vi "ELVIS III v1.0 AI Continuous Read.vi"(5 "Timeout":i32=-1 min=-1, 7 "Number of Samples":u32, 8 "error in (no error)":errorcluster, 9 "Bank Count":u8[](array[numeric]), 10 "AI (Continuous) Channels List":T1, 11 "AI (Continuous) Ref In":T3) -> (0 "error out":errorcluster, 2 "Data Output":dbl[][](array[numeric]), 3 "AI (Continuous) Ref Out":T3 caption="AI (Continuous) Ref In")   [LabVIEW 2021]
uses:
  <vilib>/myRIO/Common/Instrument Driver Framework/Utilities/typedefs/myRIO v1.0 Reference.ctl
  <vilib>/myRIO/Common/Instrument Driver Framework/Utilities/typedefs/Generic FPGA Reference.ctl
  <vilib>/myRIO/Common/Instrument Driver Framework/ELVIS III v1.0/AI Continuous/typedefs/AI Continuous Channels List.ctl
  <vilib>/myRIO/Common/Instrument Driver Framework/ELVIS III v1.0/AI Continuous/typedefs/ELVIS III v1.0 AI Continuous Channels Enum.ctl
  <vilib>/myRIO/Common/Instrument Driver Framework/ELVIS III v1.0/AI Block/typedefs/ELVIS III AI Block Channels FPGA Reference.ctl
  <vilib>/rvi/errors/niLvFpgaAdjustHostInterfaceError.vi
  <vilib>/rvi/interface/nirviReadWriteControl/nirviReadWriteControl.xnode
  <vilib>/rvi/interface/nirviMethod/nirviMethod.xnode
  <vilib>/FPGAPlugInAG/Dynamic/niLvFpga_ReadFifo_Dynamic.vi
  <vilib>/rvi/errors/niLvFpgaMergeErrorWithErrorCode.vi
  NiFpgaLv.dll
  <vilib>/rvi/interface/Simulation/niFpgaSimulationCallBeginRW.vi
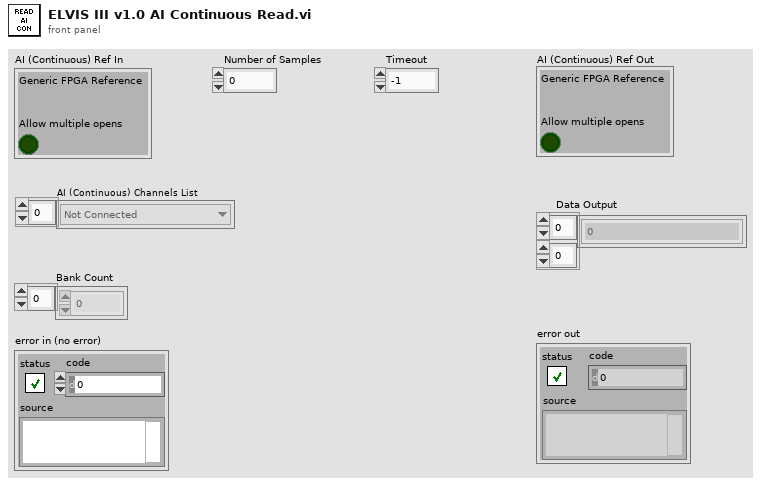
[diagram p1: front panel]
types:
  T1 = typedef "AI Continuous Channels List.ctl" = T2[]
  T2 = typedef "ELVIS III v1.0 AI Continuous Channels Enum.ctl" = enum16{"Not Connected", "A/AI0 (Continuous)", "A/AI1 (Continuous)", "A/AI2 (Continuous)", "A/AI3 (Continuous)", "A/AI4 (Continuous)", "A/AI5 (Continuous)", "A/AI6 (Continuous)", "A/AI7 (Continuous)", "A/AI0 (DIFF Continuous)", "A/AI1 (DIFF Continuous)", "A/AI2 (DIFF Continuous)", "A/AI3 (DIFF Continuous)", "B/AI0 (Continuous)", "B/AI1 (Continuous)", "B/AI2 (Continuous)", "B/AI3 (Continuous)", "B/AI4 (Continuous)", "B/AI5 (Continuous)", "B/AI6 (Continuous)", "B/AI7 (Continuous)", "B/AI0 (DIFF Continuous)", "B/AI1 (DIFF Continuous)", "B/AI2 (DIFF Continuous)", "B/AI3 (DIFF Continuous)"}
  T3 = typedef "myRIO v1.0 Reference.ctl" = cluster{"Generic FPGA Reference":T4, "Allow multiple opens":bool}
  T4 = typedef "Generic FPGA Reference.ctl" = refnum<k20>
  T5 = typedef "ELVIS III AI Block Channels FPGA Reference.ctl" = refnum<k20>
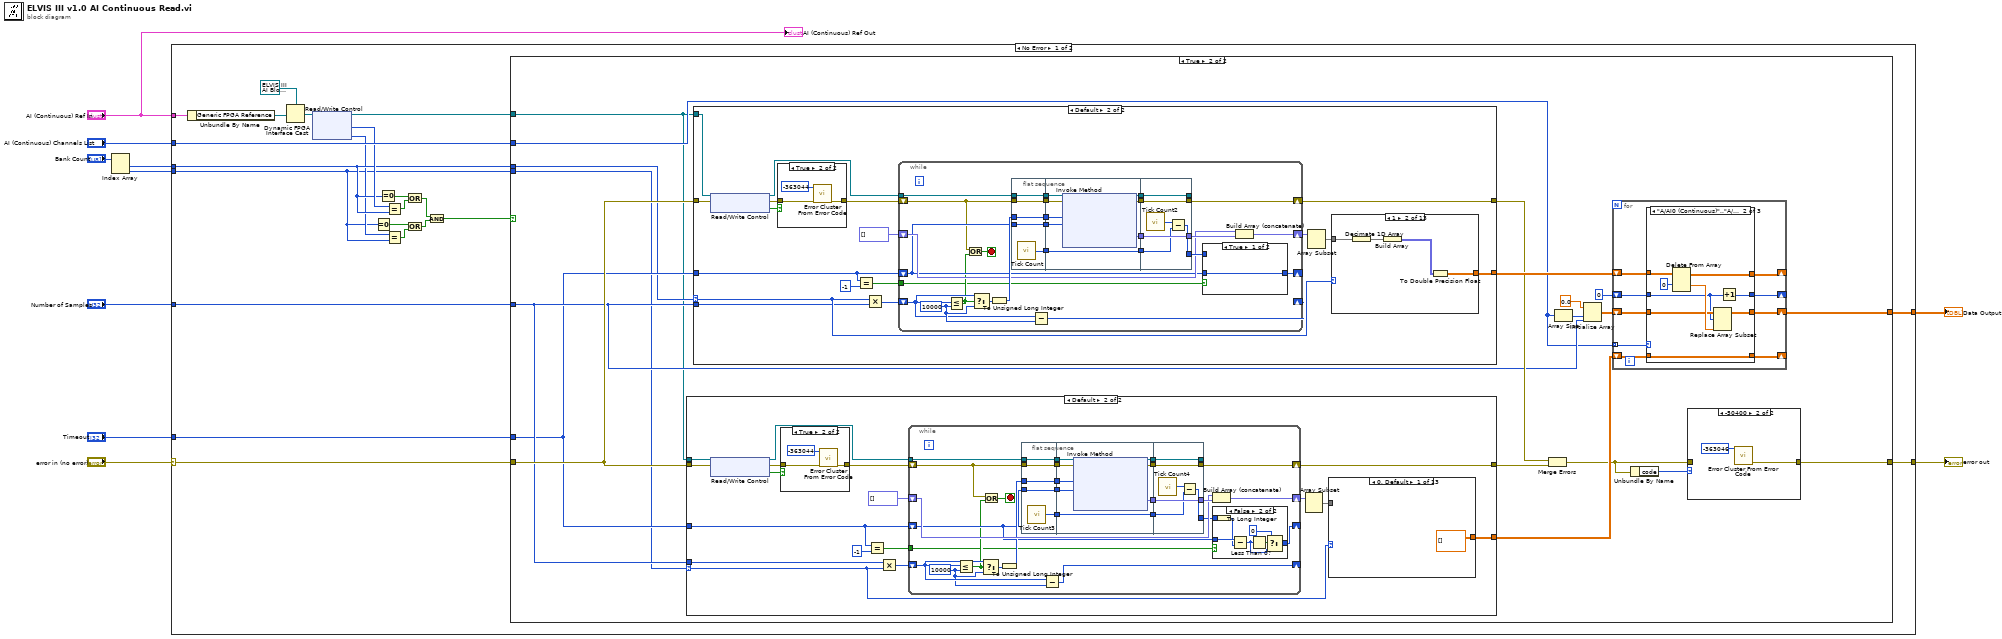
[diagram p0: block diagram]
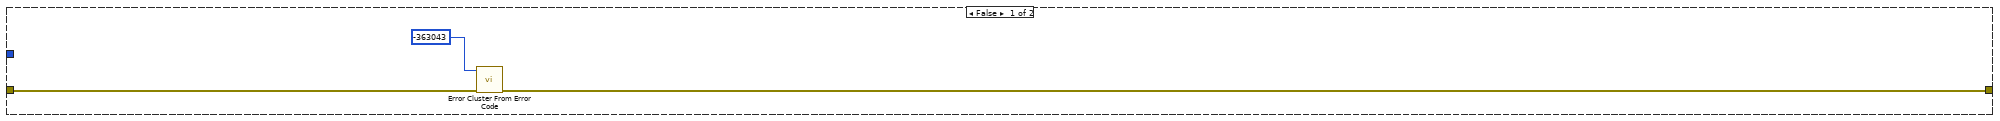
[diagram p2: hidden frame]
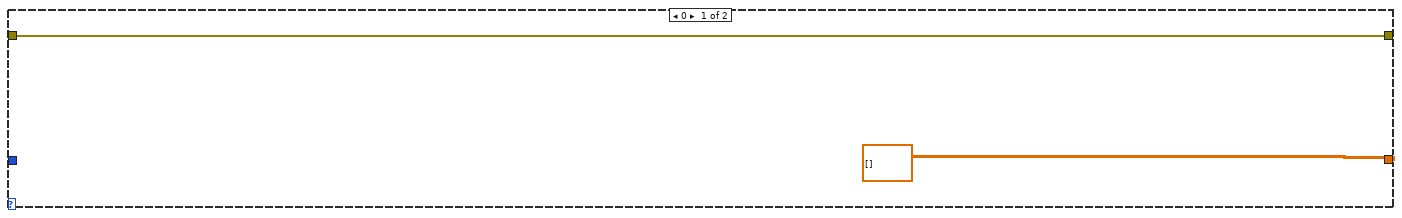
[diagram p4: hidden frame]
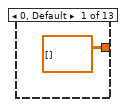
[diagram p6: hidden frame]
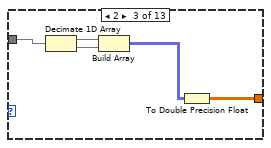
[diagram p7: hidden frame]
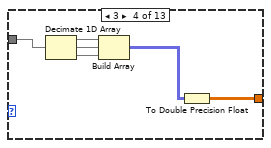
[diagram p8: hidden frame]
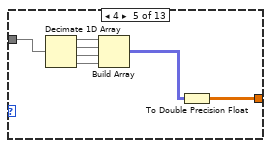
[diagram p9: hidden frame]
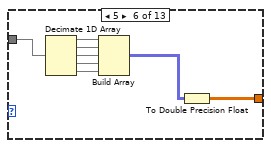
[diagram p10: hidden frame]
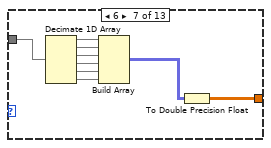
[diagram p11: hidden frame]
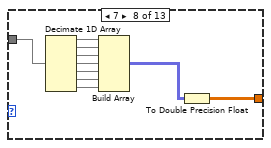
[diagram p12: hidden frame]
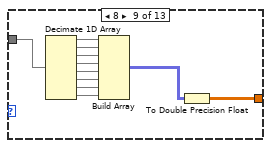
[diagram p13: hidden frame]
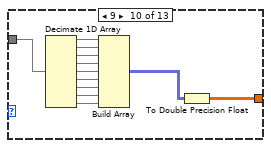
[diagram p14: hidden frame]
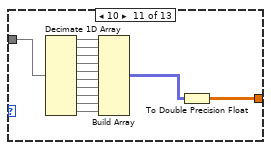
[diagram p15: hidden frame]
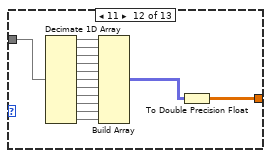
[diagram p16: hidden frame]
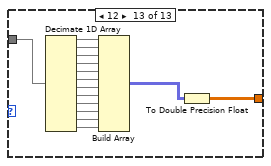
[diagram p17: hidden frame]
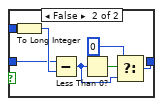
[diagram p18: hidden frame]
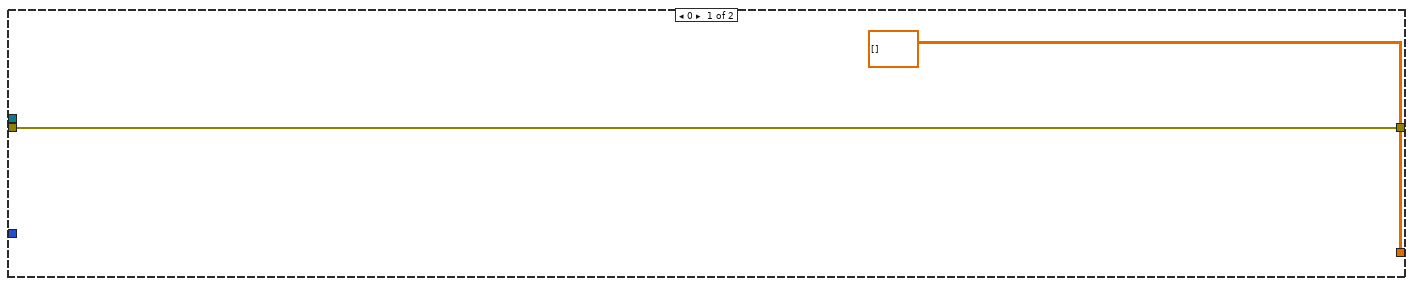
[diagram p19: hidden frame]
diagram:
  n1 = Index Array(array="Bank Count") -> (element #1=w3:u8, element #2=w2:u8)  [unwired: 2 in]
  n2 = case shown="No Error" "error in (no error)" {
    selector: "error in (no error)" -> [w30 w471]
    tunnel: "AI (Continuous) Ref In" -> [w24 _]
    tunnel: [w32 _] -> w9
    tunnel: [w31 w471] -> w8
    tunnel: "Number of Samples" -> [w29 _]
    tunnel: "Timeout" -> [w28 _]
    tunnel: w3 -> [w19 _]
    tunnel: w2 -> [w11 _]
    tunnel: "AI (Continuous) Channels List" -> [w27 _]
    frame No Error {
      n3 = Unbundle By Name(w24) -> ("Generic FPGA Reference"=w26:T4)
      n4 = Dynamic FPGA Interface Cast(Session In=T5 refnum ("AI Block Channels FPGA Reference"), Type=w26) -> (Session Out=w23:T5)
      n5 = xnode "Read/Write Control"("FPGA VI Reference In"=w23) -> ("FPGA VI Reference Out"=w22:T5, "AI.A.CNT"=w20:u8, "AI.B.CNT"=w14:u8)  [unwired: 1 in, 1 out]
      n6 = Equal To 0?(x=w11) -> (x = 0?=w15:bool)
      n7 = Equal To 0?(x=w19) -> (x = 0?=w21:bool)
      n8 = Equal?(x=w20, y=w19) -> (x = y?=w18:bool)
      n9 = Equal?(x=w14, y=w11) -> (x = y?=w16:bool)
      n10 = Or(x=w21, y=w18) -> (x .or. y?=w17:bool)
      n11 = Or(x=w15, y=w16) -> (x .or. y?=w13:bool)
      n12 = And(x=w17, y=w13) -> (x .and. y?=w12:bool)
      n13 = case shown="True" w12 {
        tunnel: [_ w46] -> w32
        tunnel: [w33 w37] -> w31
        tunnel: w30 -> [w34 w45]
        tunnel: w29 -> [_ w44]
        tunnel: w28 -> [_ w43]
        tunnel: w11 -> [_ w42]
        tunnel: w19 -> [_ w41]
        tunnel: w27 -> [_ w40]
        tunnel: w22 -> [_ w39]
        frame False {
          n14 = call <vilib>:"Error Cluster From Error Code.vi"("error in (no error)"=w34, "error code (0)"=-363043) -> ("error out"=w33:errorcluster)  [unwired: 7 in]
        }
        frame True {
          n15 = case shown="Default" w42 {
            selector: w42 -> [_ w262]
            tunnel: [dbl[][] [] w263] -> w49
            tunnel: [w250 w255] -> w47
            tunnel: w39 -> [_ w254]
            tunnel: w45 -> [w250 w253]
            tunnel: w44 -> [_ w261]
            tunnel: w43 -> [_ w259]
            frame 0 {
            }
            frame Default {
              n16 = xnode "Read/Write Control"("FPGA VI Reference In"=w254, "error in"=w253) -> ("FPGA VI Reference Out"=w251:T5, "error out"=w256:errorcluster, "AI.B.DMA_FULL"=w257:bool)
              n17 = case shown="True" w257 {
                tunnel: w256 -> [w268 w270]
                tunnel: [w268 w269] -> w252
                frame False {
                }
                frame True {
                  n18 = call <vilib>:"Error Cluster From Error Code.vi"("error in (no error)"=w270, "error code (0)"=-363044) -> ("error out"=w269:errorcluster)  [unwired: 7 in]
                }
              }
              n19 = Equal?(x=w259, y=-1) -> (x = y?=w258:bool)
              n20 = Multiply(x=w261, y=w262) -> (x*y=w267:u32)
              n21 = while {
                tunnel: w251 -> [w404]
                shift-right: [w403] -> w255
                shift-left: w252 -> [w390]
                shift-right: [w407] -> w266
                shift-left: fxp<+/-,24,5>[] [] ("Data") -> [w408]
                shift-right: [w410] -> _
                shift-left: w267 -> [w412]
                shift-right: [w391] -> _
                shift-left: w259 -> [w393]
                tunnel: w258 -> [w387]
                stop <- w388 stop-if-true
                w411 = u32 10000 ("y")
                n22 = Less Or Equal?(x=w412, y=w411) -> (x <= y?=w389:bool)
                n23 = Select(t=w412, s=w389, f=w411) -> (s? t:f=w406:u32)
                n24 = Or(x=w390, y=w389) -> (x .or. y?=w388:bool)
                n25 = To Unsigned Long Integer(number=w406) -> (unsigned 32bit integer=w405:u32)
                n26 = flat-sequence {
                  tunnel: w393 -> [w422]
                  tunnel: w390 -> [w423]
                  tunnel: w404 -> [w424]
                  tunnel: w405 -> [w425]
                  tunnel: [w425] -> w402
                  tunnel: [w424] -> w401
                  tunnel: [w423] -> w400
                  tunnel: [w422] -> w399
                  tunnel: [w421] -> w395
                  tunnel: w402 -> [w432]
                  tunnel: w401 -> [w431]
                  tunnel: w400 -> [w428]
                  tunnel: w399 -> [w427]
                  tunnel: [w433] -> w398
                  tunnel: [w430] -> w397
                  tunnel: [w429] -> w396
                  tunnel: w395 -> [w426]
                  tunnel: [w426] -> w394
                  tunnel: [w437] -> w403
                  tunnel: [w438] -> _
                  tunnel: [w439] -> w409
                  tunnel: w398 -> [w439]
                  tunnel: w397 -> [w438]
                  tunnel: w396 -> [w437]
                  tunnel: w394 -> [w436]
                  tunnel: [w435] -> w392
                  frame #0 {
                    n27 = call "Tick Count3"() -> ("Tick Count(mSec)"=w421:u32)
                  }
                  frame #1 {
                    n28 = xnode "Invoke Method"("FPGA VI Reference In"=w431, "error in"=w428, "Number of Elements"=w432, "Timeout (ms)"=w427) -> ("FPGA VI Reference Out"=w430:T5, "error out"=w429:errorcluster, "Data"=w433:fxp<+/-,24,5>[])  [unwired: 1 out]
                  }
                  frame #2 {
                    n29 = call "Tick Count4"() -> ("Tick Count(mSec)"=w434:u32)
                    n30 = Subtract(x=w434, y=w436) -> (x-y=w435:u32)
                  }
                }
                n31 = Subtract(x=w412, y=w411) -> (x-y=w410:u32)
                n32 = Build Array (concatenate)(w408, w409) -> (w407:fxp<+/-,24,5>[])
                n33 = case shown="False" w387 {
                  tunnel: w393 -> [w413 w420]
                  tunnel: w392 -> [_ w419]
                  tunnel: [w413 w414] -> w391
                  frame True {
                  }
                  frame False {
                    n34 = To Long Integer(number=w419) -> (32bit integer=w418:i32)
                    n35 = Subtract(x=w420, y=w418) -> (x-y=w416:i32)
                    n36 = Less Than 0?(x=w416) -> (x < 0?=w417:bool)
                    n37 = Select(t=0, s=w417, f=w416) -> (s? t:f=w414:i32)
                  }
                }
              }
              n38 = Array Subset(array=w266) -> (w265:fxp<+/-,24,5>[])  [unwired: 2 in]
              n39 = case shown="0, Default" w262 {
                tunnel: w265 -> [_ w276 w281 w287 w294 w302 w311 w321 w332 w344 w357 w371 w386]
                tunnel: [dbl[][] [] w274 w279 w285 w292 w300 w309 w319 w330 w342 w355 w369 w384] -> w263
                frame 0, Default {
                }
                frame 1 {
                  n40 = Decimate 1D Array(w276) -> (w275:fxp<+/-,24,5>[])
                  n41 = Build Array(w275) -> (w273:fxp<+/-,24,5>[][])
                  n42 = To Double Precision Float(number=w273) -> (double precision float=w274:dbl[][])
                }
                frame 2 {
                  n43 = Decimate 1D Array(w281) -> (w280:fxp<+/-,24,5>[], w277:fxp<+/-,24,5>[])
                  n44 = Build Array(w280, w277) -> (w278:fxp<+/-,24,5>[][])
                  n45 = To Double Precision Float(number=w278) -> (double precision float=w279:dbl[][])
                }
                frame 3 {
                  n46 = Decimate 1D Array(w287) -> (w286:fxp<+/-,24,5>[], w283:fxp<+/-,24,5>[], w282:fxp<+/-,24,5>[])
                  n47 = Build Array(w286, w283, w282) -> (w284:fxp<+/-,24,5>[][])
                  n48 = To Double Precision Float(number=w284) -> (double precision float=w285:dbl[][])
                }
                frame 4 {
                  n49 = Decimate 1D Array(w294) -> (w293:fxp<+/-,24,5>[], w290:fxp<+/-,24,5>[], w289:fxp<+/-,24,5>[], w288:fxp<+/-,24,5>[])
                  n50 = Build Array(w293, w290, w289, w288) -> (w291:fxp<+/-,24,5>[][])
                  n51 = To Double Precision Float(number=w291) -> (double precision float=w292:dbl[][])
                }
                frame 5 {
                  n52 = Decimate 1D Array(w302) -> (w301:fxp<+/-,24,5>[], w298:fxp<+/-,24,5>[], w297:fxp<+/-,24,5>[], w296:fxp<+/-,24,5>[], w295:fxp<+/-,24,5>[])
                  n53 = Build Array(w301, w298, w297, w296, w295) -> (w299:fxp<+/-,24,5>[][])
                  n54 = To Double Precision Float(number=w299) -> (double precision float=w300:dbl[][])
                }
                frame 6 {
                  n55 = Decimate 1D Array(w311) -> (w310:fxp<+/-,24,5>[], w307:fxp<+/-,24,5>[], w306:fxp<+/-,24,5>[], w305:fxp<+/-,24,5>[], w304:fxp<+/-,24,5>[], w303:fxp<+/-,24,5>[])
                  n56 = Build Array(w310, w307, w306, w305, w304, w303) -> (w308:fxp<+/-,24,5>[][])
                  n57 = To Double Precision Float(number=w308) -> (double precision float=w309:dbl[][])
                }
                frame 7 {
                  n58 = Decimate 1D Array(w321) -> (w320:fxp<+/-,24,5>[], w317:fxp<+/-,24,5>[], w316:fxp<+/-,24,5>[], w315:fxp<+/-,24,5>[], w314:fxp<+/-,24,5>[], w313:fxp<+/-,24,5>[], w312:fxp<+/-,24,5>[])
                  n59 = Build Array(w320, w317, w316, w315, w314, w313, w312) -> (w318:fxp<+/-,24,5>[][])
                  n60 = To Double Precision Float(number=w318) -> (double precision float=w319:dbl[][])
                }
                frame 8 {
                  n61 = Decimate 1D Array(w332) -> (w331:fxp<+/-,24,5>[], w328:fxp<+/-,24,5>[], w327:fxp<+/-,24,5>[], w326:fxp<+/-,24,5>[], w325:fxp<+/-,24,5>[], w324:fxp<+/-,24,5>[], w323:fxp<+/-,24,5>[], w322:fxp<+/-,24,5>[])
                  n62 = Build Array(w331, w328, w327, w326, w325, w324, w323, w322) -> (w329:fxp<+/-,24,5>[][])
                  n63 = To Double Precision Float(number=w329) -> (double precision float=w330:dbl[][])
                }
                frame 9 {
                  n64 = Decimate 1D Array(w344) -> (w343:fxp<+/-,24,5>[], w340:fxp<+/-,24,5>[], w339:fxp<+/-,24,5>[], w338:fxp<+/-,24,5>[], w337:fxp<+/-,24,5>[], w336:fxp<+/-,24,5>[], w335:fxp<+/-,24,5>[], w334:fxp<+/-,24,5>[], w333:fxp<+/-,24,5>[])
                  n65 = Build Array(w343, w340, w339, w338, w337, w336, w335, w334, w333) -> (w341:fxp<+/-,24,5>[][])
                  n66 = To Double Precision Float(number=w341) -> (double precision float=w342:dbl[][])
                }
                frame 10 {
                  n67 = Decimate 1D Array(w357) -> (w356:fxp<+/-,24,5>[], w353:fxp<+/-,24,5>[], w352:fxp<+/-,24,5>[], w351:fxp<+/-,24,5>[], w350:fxp<+/-,24,5>[], w349:fxp<+/-,24,5>[], w348:fxp<+/-,24,5>[], w347:fxp<+/-,24,5>[], w346:fxp<+/-,24,5>[], w345:fxp<+/-,24,5>[])
                  n68 = Build Array(w356, w353, w352, w351, w350, w349, w348, w347, w346, w345) -> (w354:fxp<+/-,24,5>[][])
                  n69 = To Double Precision Float(number=w354) -> (double precision float=w355:dbl[][])
                }
                frame 11 {
                  n70 = Decimate 1D Array(w371) -> (w370:fxp<+/-,24,5>[], w367:fxp<+/-,24,5>[], w366:fxp<+/-,24,5>[], w365:fxp<+/-,24,5>[], w364:fxp<+/-,24,5>[], w363:fxp<+/-,24,5>[], w362:fxp<+/-,24,5>[], w361:fxp<+/-,24,5>[], w360:fxp<+/-,24,5>[], w359:fxp<+/-,24,5>[], w358:fxp<+/-,24,5>[])
                  n71 = Build Array(w370, w367, w366, w365, w364, w363, w362, w361, w360, w359, w358) -> (w368:fxp<+/-,24,5>[][])
                  n72 = To Double Precision Float(number=w368) -> (double precision float=w369:dbl[][])
                }
                frame 12 {
                  n73 = Decimate 1D Array(w386) -> (w385:fxp<+/-,24,5>[], w382:fxp<+/-,24,5>[], w381:fxp<+/-,24,5>[], w380:fxp<+/-,24,5>[], w379:fxp<+/-,24,5>[], w378:fxp<+/-,24,5>[], w377:fxp<+/-,24,5>[], w376:fxp<+/-,24,5>[], w375:fxp<+/-,24,5>[], w374:fxp<+/-,24,5>[], w373:fxp<+/-,24,5>[], w372:fxp<+/-,24,5>[])
                  n74 = Build Array(w385, w382, w381, w380, w379, w378, w377, w376, w375, w374, w373, w372) -> (w383:fxp<+/-,24,5>[][])
                  n75 = To Double Precision Float(number=w383) -> (double precision float=w384:dbl[][])
                }
              }
            }
          }
          n76 = case shown="Default" w41 {
            selector: w41 -> [_ w71]
            tunnel: [dbl[][] [] w72] -> w50
            tunnel: [w59 w64] -> w48
            tunnel: w39 -> [_ w61]
            tunnel: w45 -> [w59 w63]
            tunnel: w44 -> [_ w70]
            tunnel: w43 -> [_ w69]
            frame 0 {
            }
            frame Default {
              n77 = xnode "Read/Write Control"("FPGA VI Reference In"=w61, "error in"=w63) -> ("FPGA VI Reference Out"=w60:T5, "error out"=w66:errorcluster, "AI.A.DMA_FULL"=w65:bool)
              n78 = case shown="True" w65 {
                tunnel: w66 -> [w77 w79]
                tunnel: [w77 w78] -> w62
                frame False {
                }
                frame True {
                  n79 = call <vilib>:"Error Cluster From Error Code.vi"("error in (no error)"=w79, "error code (0)"=-363044) -> ("error out"=w78:errorcluster)  [unwired: 7 in]
                }
              }
              n80 = Equal?(x=w69, y=-1) -> (x = y?=w67:bool)
              n81 = Multiply(x=w71, y=w70) -> (x*y=w73:u32)
              n82 = while {
                tunnel: w60 -> [w210]
                shift-right: [w208] -> w64
                shift-left: w62 -> [w199]
                shift-right: [w207] -> w74
                shift-left: fxp<+/-,24,5>[] [] ("Data") -> [w206]
                shift-right: [w200] -> _
                shift-left: w73 -> [w201]
                shift-right: [w203] -> _
                shift-left: w69 -> [w204]
                tunnel: w67 -> [w196]
                stop <- w197 stop-if-true
                w202 = u32 10000 ("y")
                n83 = Less Or Equal?(x=w201, y=w202) -> (x <= y?=w198:bool)
                n84 = Or(x=w199, y=w198) -> (x .or. y?=w197:bool)
                n85 = Select(t=w201, s=w198, f=w202) -> (s? t:f=w221:u32)
                n86 = To Unsigned Long Integer(number=w221) -> (unsigned 32bit integer=w212:u32)
                n87 = flat-sequence {
                  tunnel: w212 -> [w234]
                  tunnel: [w234] -> w220
                  tunnel: [w230] -> w219
                  tunnel: w199 -> [w233]
                  tunnel: [w233] -> w211
                  tunnel: w210 -> [w232]
                  tunnel: [w232] -> w209
                  tunnel: w204 -> [w231]
                  tunnel: [w231] -> w205
                  tunnel: w220 -> [w241]
                  tunnel: [w242] -> w218
                  tunnel: [w240] -> w217
                  tunnel: [w239] -> w216
                  tunnel: w219 -> [w238]
                  tunnel: [w238] -> w215
                  tunnel: w211 -> [w237]
                  tunnel: w209 -> [w236]
                  tunnel: w205 -> [w235]
                  tunnel: [w246] -> w208
                  tunnel: [w247] -> _
                  tunnel: [w248] -> w214
                  tunnel: w218 -> [w248]
                  tunnel: w217 -> [w247]
                  tunnel: w216 -> [w246]
                  tunnel: w215 -> [w245]
                  tunnel: [w244] -> w213
                  frame #0 {
                    n88 = call "Tick Count"() -> ("Tick Count(mSec)"=w230:u32)
                  }
                  frame #1 {
                    n89 = xnode "Invoke Method"("FPGA VI Reference In"=w236, "error in"=w237, "Number of Elements"=w241, "Timeout (ms)"=w235) -> ("FPGA VI Reference Out"=w240:T5, "error out"=w239:errorcluster, "Data"=w242:fxp<+/-,24,5>[])  [unwired: 1 out]
                  }
                  frame #2 {
                    n90 = call "Tick Count2"() -> ("Tick Count(mSec)"=w243:u32)
                    n91 = Subtract(x=w243, y=w245) -> (x-y=w244:u32)
                  }
                }
                n92 = Subtract(x=w201, y=w202) -> (x-y=w200:u32)
                n93 = case shown="True" w196 {
                  tunnel: w213 -> [_ w229]
                  tunnel: w204 -> [w222 w224]
                  tunnel: [w222 w223] -> w203
                  frame True {
                  }
                  frame False {
                    n94 = To Long Integer(number=w229) -> (32bit integer=w228:i32)
                    n95 = Subtract(x=w224, y=w228) -> (x-y=w226:i32)
                    n96 = Less Than 0?(x=w226) -> (x < 0?=w227:bool)
                    n97 = Select(t=0, s=w227, f=w226) -> (s? t:f=w223:i32)
                  }
                }
                n98 = Build Array (concatenate)(w206, w214) -> (w207:fxp<+/-,24,5>[])
              }
              n99 = Array Subset(array=w74) -> (w75:fxp<+/-,24,5>[])  [unwired: 2 in]
              n100 = case shown="1" w71 {
                tunnel: w75 -> [_ w85 w90 w96 w103 w111 w120 w130 w141 w153 w166 w180 w195]
                tunnel: [dbl[][] [] w83 w88 w94 w101 w109 w118 w128 w139 w151 w164 w178 w193] -> w72
                frame 0, Default {
                }
                frame 1 {
                  n101 = Decimate 1D Array(w85) -> (w84:fxp<+/-,24,5>[])
                  n102 = Build Array(w84) -> (w82:fxp<+/-,24,5>[][])
                  n103 = To Double Precision Float(number=w82) -> (double precision float=w83:dbl[][])
                }
                frame 2 {
                  n104 = Decimate 1D Array(w90) -> (w89:fxp<+/-,24,5>[], w86:fxp<+/-,24,5>[])
                  n105 = Build Array(w89, w86) -> (w87:fxp<+/-,24,5>[][])
                  n106 = To Double Precision Float(number=w87) -> (double precision float=w88:dbl[][])
                }
                frame 3 {
                  n107 = Decimate 1D Array(w96) -> (w95:fxp<+/-,24,5>[], w92:fxp<+/-,24,5>[], w91:fxp<+/-,24,5>[])
                  n108 = Build Array(w95, w92, w91) -> (w93:fxp<+/-,24,5>[][])
                  n109 = To Double Precision Float(number=w93) -> (double precision float=w94:dbl[][])
                }
                frame 4 {
                  n110 = Decimate 1D Array(w103) -> (w102:fxp<+/-,24,5>[], w99:fxp<+/-,24,5>[], w98:fxp<+/-,24,5>[], w97:fxp<+/-,24,5>[])
                  n111 = Build Array(w102, w99, w98, w97) -> (w100:fxp<+/-,24,5>[][])
                  n112 = To Double Precision Float(number=w100) -> (double precision float=w101:dbl[][])
                }
                frame 5 {
                  n113 = Decimate 1D Array(w111) -> (w110:fxp<+/-,24,5>[], w107:fxp<+/-,24,5>[], w106:fxp<+/-,24,5>[], w105:fxp<+/-,24,5>[], w104:fxp<+/-,24,5>[])
                  n114 = Build Array(w110, w107, w106, w105, w104) -> (w108:fxp<+/-,24,5>[][])
                  n115 = To Double Precision Float(number=w108) -> (double precision float=w109:dbl[][])
                }
                frame 6 {
                  n116 = Decimate 1D Array(w120) -> (w119:fxp<+/-,24,5>[], w116:fxp<+/-,24,5>[], w115:fxp<+/-,24,5>[], w114:fxp<+/-,24,5>[], w113:fxp<+/-,24,5>[], w112:fxp<+/-,24,5>[])
                  n117 = Build Array(w119, w116, w115, w114, w113, w112) -> (w117:fxp<+/-,24,5>[][])
                  n118 = To Double Precision Float(number=w117) -> (double precision float=w118:dbl[][])
                }
                frame 7 {
                  n119 = Decimate 1D Array(w130) -> (w129:fxp<+/-,24,5>[], w126:fxp<+/-,24,5>[], w125:fxp<+/-,24,5>[], w124:fxp<+/-,24,5>[], w123:fxp<+/-,24,5>[], w122:fxp<+/-,24,5>[], w121:fxp<+/-,24,5>[])
                  n120 = Build Array(w129, w126, w125, w124, w123, w122, w121) -> (w127:fxp<+/-,24,5>[][])
                  n121 = To Double Precision Float(number=w127) -> (double precision float=w128:dbl[][])
                }
                frame 8 {
                  n122 = Decimate 1D Array(w141) -> (w140:fxp<+/-,24,5>[], w137:fxp<+/-,24,5>[], w136:fxp<+/-,24,5>[], w135:fxp<+/-,24,5>[], w134:fxp<+/-,24,5>[], w133:fxp<+/-,24,5>[], w132:fxp<+/-,24,5>[], w131:fxp<+/-,24,5>[])
                  n123 = Build Array(w140, w137, w136, w135, w134, w133, w132, w131) -> (w138:fxp<+/-,24,5>[][])
                  n124 = To Double Precision Float(number=w138) -> (double precision float=w139:dbl[][])
                }
                frame 9 {
                  n125 = Decimate 1D Array(w153) -> (w152:fxp<+/-,24,5>[], w149:fxp<+/-,24,5>[], w148:fxp<+/-,24,5>[], w147:fxp<+/-,24,5>[], w146:fxp<+/-,24,5>[], w145:fxp<+/-,24,5>[], w144:fxp<+/-,24,5>[], w143:fxp<+/-,24,5>[], w142:fxp<+/-,24,5>[])
                  n126 = Build Array(w152, w149, w148, w147, w146, w145, w144, w143, w142) -> (w150:fxp<+/-,24,5>[][])
                  n127 = To Double Precision Float(number=w150) -> (double precision float=w151:dbl[][])
                }
                frame 10 {
                  n128 = Decimate 1D Array(w166) -> (w165:fxp<+/-,24,5>[], w162:fxp<+/-,24,5>[], w161:fxp<+/-,24,5>[], w160:fxp<+/-,24,5>[], w159:fxp<+/-,24,5>[], w158:fxp<+/-,24,5>[], w157:fxp<+/-,24,5>[], w156:fxp<+/-,24,5>[], w155:fxp<+/-,24,5>[], w154:fxp<+/-,24,5>[])
                  n129 = Build Array(w165, w162, w161, w160, w159, w158, w157, w156, w155, w154) -> (w163:fxp<+/-,24,5>[][])
                  n130 = To Double Precision Float(number=w163) -> (double precision float=w164:dbl[][])
                }
                frame 11 {
                  n131 = Decimate 1D Array(w180) -> (w179:fxp<+/-,24,5>[], w176:fxp<+/-,24,5>[], w175:fxp<+/-,24,5>[], w174:fxp<+/-,24,5>[], w173:fxp<+/-,24,5>[], w172:fxp<+/-,24,5>[], w171:fxp<+/-,24,5>[], w170:fxp<+/-,24,5>[], w169:fxp<+/-,24,5>[], w168:fxp<+/-,24,5>[], w167:fxp<+/-,24,5>[])
                  n132 = Build Array(w179, w176, w175, w174, w173, w172, w171, w170, w169, w168, w167) -> (w177:fxp<+/-,24,5>[][])
                  n133 = To Double Precision Float(number=w177) -> (double precision float=w178:dbl[][])
                }
                frame 12 {
                  n134 = Decimate 1D Array(w195) -> (w194:fxp<+/-,24,5>[], w191:fxp<+/-,24,5>[], w190:fxp<+/-,24,5>[], w189:fxp<+/-,24,5>[], w188:fxp<+/-,24,5>[], w187:fxp<+/-,24,5>[], w186:fxp<+/-,24,5>[], w185:fxp<+/-,24,5>[], w184:fxp<+/-,24,5>[], w183:fxp<+/-,24,5>[], w182:fxp<+/-,24,5>[], w181:fxp<+/-,24,5>[])
                  n135 = Build Array(w194, w191, w190, w189, w188, w187, w186, w185, w184, w183, w182, w181) -> (w192:fxp<+/-,24,5>[][])
                  n136 = To Double Precision Float(number=w192) -> (double precision float=w193:dbl[][])
                }
              }
            }
          }
          n137 = Merge Errors(w48, w47) -> (w36:errorcluster)
          n138 = Array Size(array=w40) -> (size(s)=w54:i32)
          n139 = Initialize Array(0.0, w54, w44) -> (w51:dbl[][])
          n140 = for {
            tunnel: w40 -> [w448] mode=indexing
            shift-right: [w445] -> _
            shift-left: w50 -> [w447]
            shift-right: [w440] -> w46
            shift-left: w51 -> [w443]
            shift-right: [w444] -> _
            shift-left: w49 -> [w446]
            shift-right: [w441] -> _
            shift-left: 0 -> [w442]
            n141 = case shown="\"A/AI0 (Continuous)\"..\"A/AI3 (DIFF Continuous)\"" w448 {
              tunnel: w447 -> [w452 w461 w468]
              tunnel: [w452 w459 w468] -> w445
              tunnel: w446 -> [w451 w458 w469]
              tunnel: [w451 w458 w467] -> w444
              tunnel: w443 -> [w449 w456 w466]
              tunnel: w442 -> [w450 w455 w463]
              tunnel: [w450 w454 w462] -> w441
              tunnel: [w449 w453 w465] -> w440
              frame "Not Connected", Default {
              }
              frame "A/AI0 (Continuous)".."A/AI3 (DIFF Continuous)" {
                n142 = Delete From Array(array=w461, index (row)=0) -> (deleted portion=w457:dbl[], array with subset deleted=w459:dbl[][])  [unwired: 2 in]
                n143 = Replace Array Subset(array=w456, new element=w457, index (row)=w455) -> (w453:dbl[][])  [unwired: 1 in]
                n144 = Increment(x=w455) -> (x+1=w454:i32)
              }
              frame "B/AI0 (Continuous)".."B/AI3 (DIFF Continuous)" {
                n145 = Delete From Array(array=w469, index (row)=0) -> (deleted portion=w464:dbl[], array with subset deleted=w467:dbl[][])  [unwired: 2 in]
                n146 = Replace Array Subset(array=w466, new element=w464, index (row)=w463) -> (w465:dbl[][])  [unwired: 1 in]
                n147 = Increment(x=w463) -> (x+1=w462:i32)
              }
            }
          }
          n148 = Unbundle By Name(w36) -> ("code"=w38:i32)
          n149 = case shown="-50400" w38 {
            tunnel: [w55 w56] -> w37
            tunnel: w36 -> [w55 _]
            frame Default {
            }
            frame -50400 {
              n150 = call <vilib>:"Error Cluster From Error Code.vi"("error code (0)"=-363046) -> ("error out"=w56:errorcluster)  [unwired: 8 in]
            }
          }
        }
      }
    }
    frame Error {
    }
  }
  "error out" <- w8
  "Data Output" <- w9
  "AI (Continuous) Ref Out" <- "AI (Continuous) Ref In"
